vi "Measurement_Measure_StreamsExpectedResults.vi"(8 "error in":errorcluster, 11 "run service vi":refnum<vi>) -> (0 "error out":errorcluster, 2 "result":string, 3 "pass":bool)   [LabVIEW 2021, in "MeasurementServerTests.lvlib" / "Measurement Service Tests.lvlib"]
uses:
  Measurement Service Tests.lvlib
  Runtime/Measurements/Helpers/TypeDefs/Measurement Server User Settings.ctl
  Runtime/Measurements/Helpers/TypeDefs/Stop Server User Event.ctl
  Runtime/Measurements/Helpers/TypeDefs/Measurement Service Version.ctl
  Continuous Counting Client/controls/Measurement Configuration.ctl
  5197d96a-511e-46f8-85e2-3078f9cd6078.vi
  Runtime/Measurements/NI Measurement Plug-In SDK.lvlib
  Continuous Counting Client/Continuous Counting Client.lvlib
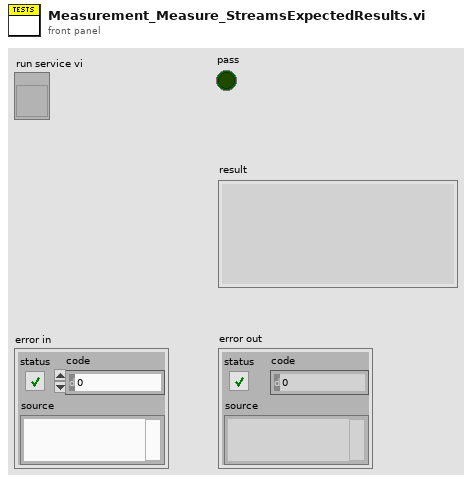
[diagram p1: front panel]
types:
  T1 = typedef "MeasurementServerTests.lvlib/Measurement Service Tests.lvlib/Continuous Counting Client.lvlib/Measurement Configuration.ctl" = cluster{"ms update interval":u32}
  T2 = typedef "NI Measurement Plug-In SDK.lvlib/Measurement Service Version.ctl" = enum16{"V1", "V2"}
  T3 = typedef "NI Measurement Plug-In SDK.lvlib/Measurement Server User Settings.ctl" = cluster{"stop server":T4, "measurement service versions":T2[]}
  T4 = typedef "NI Measurement Plug-In SDK.lvlib/Stop Server User Event.ctl" = refnum<user-event>
  T5 = typedef "grpc-lvsupport-release.lvlib/grpcId.ctl" = u64
  T6 = typedef "MeasurementServerTests.lvlib/Measurement Service Tests.lvlib/Continuous Counting Client.lvlib/Measurement Results.ctl" = cluster{"current count":i64}
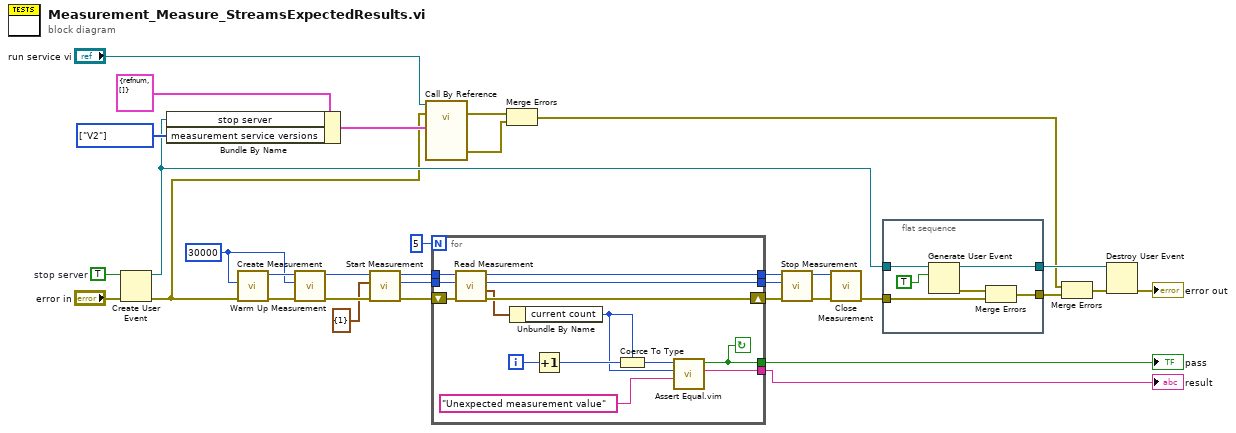
[diagram p0: block diagram]
diagram:
  w22 = 30000 ("ms timeout")
  w31 = TRUE  # stop server
  w32 = T2[] [enum."V2"] items=["V1", "V2"] ("measurement service versions")
  n1 = Create User Event(user event datatype=w31, error in="error in") -> (user event=w29:refnum<user-event>, error out=w4:errorcluster)
  n2 = Bundle By Name(cluster=T3 {"stop server"=refnum, "measurement service versions"=[]} ("server settings"), "stop server"=w29, "measurement service versions"=w32) -> (w5:T3)
  n3 = call "Create Measurement.vi"("error in"=w4, "ms timeout"=w22) -> ("error out"=w26:errorcluster, "gRPCid out"=w23:T5)  [unwired: 8 in]
  n4 = call "Warm Up Measurement.vi"("error in"=w26, "timeout (ms)"=w22, "gRPC ID"=w23) -> ("error out"=w25:errorcluster, "gRPC ID out"=w24:T5)  [unwired: 6 in, 1 out]
  n5 = call "Start Measurement.vi"("error in"=w25, "measurement configuration"=T1 {"ms update interval"=1}, "gRPCid in"=w24) -> ("error out"=w16:errorcluster, "call id"=w15:T5, "gRPCid out"=w17:T5)  [unwired: 6 in]
  n6 = call-by-ref "?"(reference="run service vi", error in=w4, "server settings"=w5) -> (error out=w6:errorcluster, 0:"error out"=w1:errorcluster)  [unwired: 10 in, 1 out]
  n7 = for {
    N: 5 -> [_]
    tunnel: w17 -> [w47]
    tunnel: w15 -> [w45]
    tunnel: [w44] -> w14
    tunnel: [w43] -> w13
    shift-right: [w42] -> w11
    shift-left: w16 -> [w46]
    tunnel: [w39] -> w7
    tunnel: [w38] -> w8
    i -> [w40]
    stop <- w39 continue-if-true
    n8 = call "Read Measurement.vi"("error in"=w46, "call id in"=w45, "gRPCid in"=w47) -> ("error out"=w42:errorcluster, "measurement results"=w41:T6, "call id out"=w44:T5, "gRPCid out"=w43:T5)  [unwired: 4 in, 1 out]
    n9 = Unbundle By Name(w41) -> ("current count"=w34:i64)
    n10 = Increment(x=w40) -> (x+1=w36:i32)
    n11 = Coerce To Type(0:w36, 1:w34) -> (2:w35:i64)
    n12 = call "Assert Equal.vim"("failure message"="Unexpected measurement value", "actual value"=w34, "expected value"=w35) -> ("message"=w38:string, "equal?"=w39:bool)  [unwired: 7 in]
  }
  "pass" <- w7
  "result" <- w8
  n13 = Merge Errors(w6, w1) -> (w2:errorcluster)
  n14 = call "Stop Measurement.vi"("error in"=w11, "call id"=w14, "gRPCid in"=w13) -> ("error out"=w12:errorcluster, "gRPCid out"=w27:T5)  [unwired: 7 in]
  n15 = call "Close Measurement.vi"("error in"=w12, "gRPCid in"=w27) -> ("error out"=w28:errorcluster)  [unwired: 9 in]
  n16 = flat-sequence {
    tunnel: w29 -> [w52]
    tunnel: [w51] -> w19
    tunnel: [w50] -> w21
    tunnel: w28 -> [w49]
    frame #0 {
      n17 = Generate User Event(user event=w52, event data cluster=TRUE ("event data")) -> (user event out=w51:refnum<user-event>, error out=w53:errorcluster)  [unwired: 2 in]
      n18 = Merge Errors(w53, w49) -> (w50:errorcluster)
    }
  }
  n19 = Merge Errors(w2, w21) -> (w20:errorcluster)
  n20 = Destroy User Event(user event=w19, error in=w20) -> (error out=→"error out":errorcluster)
